vi "Receiver_Example - 2 Channel - Experiment_7.vi"() -> ()   [LabVIEW 2022 SP3]
panel:
  out "x = 0?":bool
  out "iterationsIM":dbl
  in  "State":i32
  in  "Counter":dbl
  in  "OFDM - 4QAM/16QAM":bool
  out "Iterations 2":i32
  in  "Tab Control 3":enum32{"OFDM - 4QAM", "16QAM"}(tab)
  in  "Tab Control":enum32{"USRP Parameters", "Rx Info", "BER"}(tab)
  in  "USRP ControledParameters":T1={"Active Antenna"="RX2", "Gain (dB)"=10.0, "Carrier Frequency"=2400000000.0, "IQ Rate"=2000000.0, "Active channels"="0,1"} {"IQ Rate" format="%#_6p"; "Carrier Frequency" format="%#_6p"; "Gain (dB)" format="%#_6f"}
  in  "Device selection":refnum<k15>="RIO0"
  in  "Trigger level":dbl=0.005 format="%f"
  out "CH0":T2
  out "CH1":T2
  out "SIG valid? - CH1":bool
  out "SIG valid? - CH0":bool
  out "Frequency offset - CH1":dbl
  out "Frequency offset - CH0":dbl
  out "Coerced Parameters":T3={"IQ Rate"=100000.0, "Carrier  Freq."=100000.0, "Gain"=0.0} {"Gain" format="%#_6f"; "Carrier  Freq." format="%#_6p"; "IQ Rate" format="%#_6p"}
  out "Error out":errorcluster
  in  "Expected message LP - CH0":string="Non Critical Data\nNon Critical Data\nNon Critical Data\nNon Critical Data\nNon Critical Data"
  in  "Expected message - CH1":string="Critical Dataaaaa\nCritical Dataaaaa\nCritical Dataaaaa\nCritical Dataaaaa\nCritical Dataaaaa"
  out "Expected message LP Detected CH0":string="Non Critical Data\nNon Critical Data\nNon Critical Data\nNon Critical Data\nNon Critical Data"
  out "Expected message HP Detected CH1":string="Non Critical Data\nNon Critical Data\nNon Critical Data\nNon Critical Data\nNon Critical Data"
  in  "Boolean":bool
  in  "Boolean 3":bool
  out "Expected message HP Detected CH0":string="Non Critical Data\nNon Critical Data\nNon Critical Data\nNon Critical Data\nNon Critical Data"
  in  "Expected message HP - CH0":string="Critical Dataaaaa\nCritical Dataaaaa\nCritical Dataaaaa\nCritical Dataaaaa\nCritical Dataaaaa"
  in  "Boolean 2":bool
  out "Inst. BER HP - CH0":dbl format="%#_4g"
  out "Acc. BER HP - CH0":dbl format="%#_4g"
  out "Acum. Err HP - CH0":dbl
  out "No. Bits HP - CH0":dbl
  out "Acc. BER LP - CH0":dbl format="%#_4g"
  out "Inst. BER - CH1":dbl format="%#_4g"
  out "Inst. BER LP - CH0":dbl format="%#_4g"
  out "No. Bits - CH1":dbl
  out "No. Bits LP - CH0":dbl
  out "Acum. Err - CH1":dbl
  out "Acum. Err LP - CH0":dbl
  in  "Record BER":bool
  in  "Refresh Button":bool
  out "Acc. BER - CH1":dbl format="%#_4g"
  in  "Low-Power Window Size - CH0":dbl=15.0 format="%#_6p"
  in  "High-Power Window Size":dbl=15.0 format="%#_6p"
  out "High-Power Image 2":T4(plugin-control)
  in  "Tab Control 2":enum32{"1 Channel", "2 Channel"}(tab)
  in  "Save data 1 channel":bool
  out "Constellation Map 1 Channel":cdb[](graph)
  out "Low-Power BER - 1 Channel":dbl(graph)
  out "High-Power BER - 1 Channel":dbl(graph)
  out "High-Power Decoded message - 1 Channel":string
  out "Low-Power Decoded message - 1 Channel":string
  out "Low-Power Decoded message - CH0":string
  out "Decoded message - CH1":string
  out "Constellation Map 2 Channel":cluster{"Constellation":cdb[]}[](graph)
  out "Low-Power BER - CH0":dbl(graph)
  out "High-Power BER":T5(graph)
  out "High-Power Decoded message - CH0":string
  out "CH1 2":bool
  out "CH0 2":bool
  in  "Save data 2 channels":bool
  in  "Channel":bool
  in  "Save data":bool
  out "Reconstructed Image":T4(plugin-control)
  out "Expected message  HP  Detected 2":string="Critical Dataaaaa\nCritical Dataaaaa\nCritical Dataaaaa\nCritical Dataaaaa\nCritical Dataaaaa"
  in  "Boolean 4":bool
  in  "High-Power Window Size 2":dbl=15.0 format="%#_6p"
  out "High-Power Instantaneous BER Graph 2":u8(slide) scale=0.0..100.0
  out "High-Power BER Graph 2":dbl(graph)
  out "No. Bits HP 2":dbl
  out "Acc. BER  HP 2":dbl format="%#_4g"
  out "Acum. Err HP 2":dbl
  out "Inst. BER HP 2":dbl format="%#_4g"
  in  "Expected message 2 HP 2":string="Critical Dataaaaa\nCritical Dataaaaa\nCritical Dataaaaa\nCritical Dataaaaa\nCritical Dataaaaa"
  out "High-Power Decoded Message 2":string
  in  "Record BER 2":bool
  out "Constellation Map 2":cdb[](graph)
  out "Frequency offset 2":dbl
  out "SIG valid? 2":bool
  in  "Refresh Button 2":bool
  out "Error out 2":errorcluster
  in  "error in (no error)":errorcluster
  # "OFDM Superposition Coded Receiver"
  # "1 Channel"
  # "2 Channel"
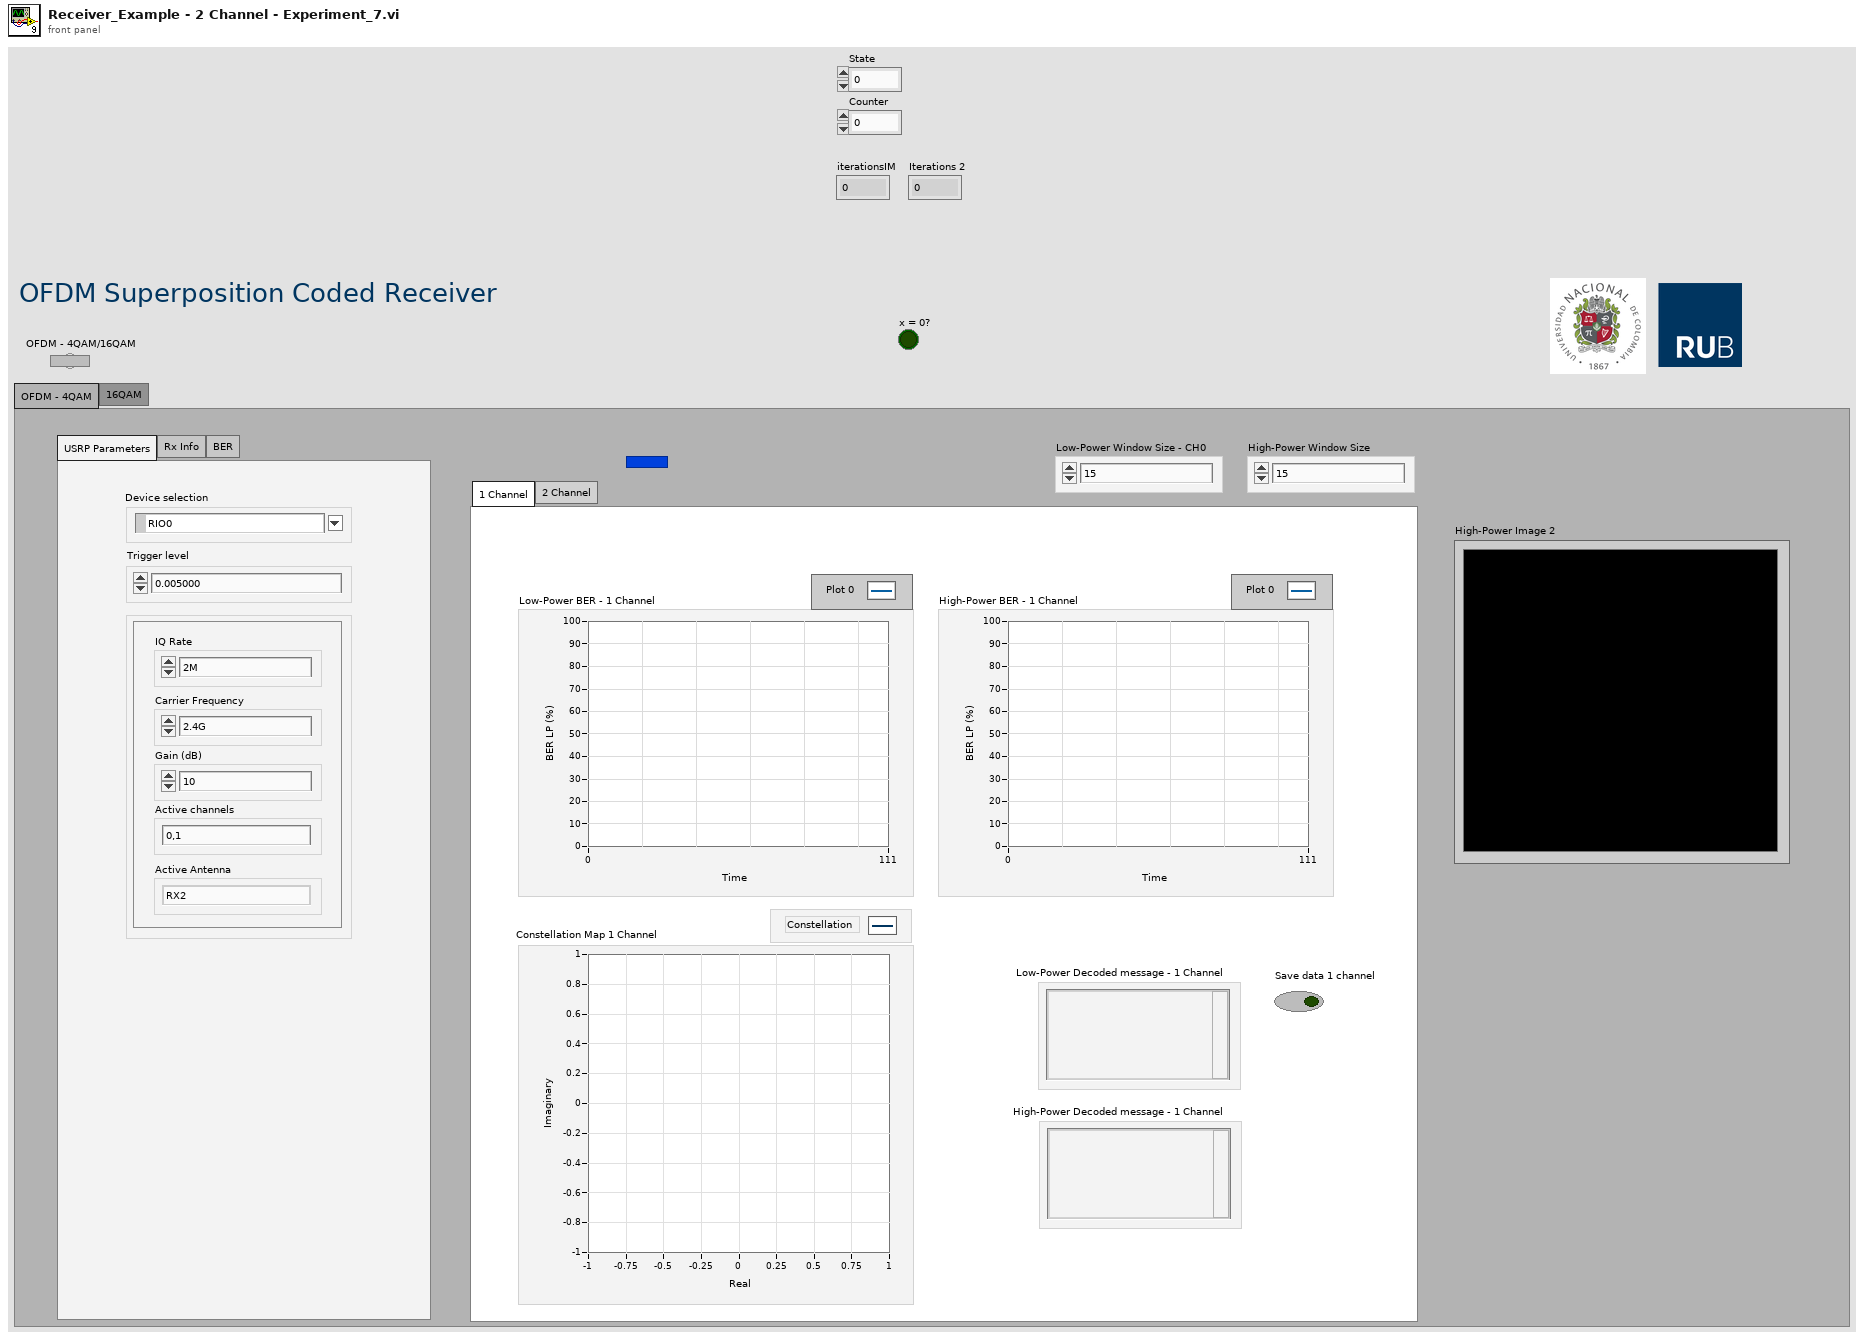
[diagram p1: front panel]
types:
  T1 = cluster{"Active Antenna":string, "Gain (dB)":dbl, "Carrier Frequency":dbl, "IQ Rate":dbl, "Active channels":string}
  T2 = cluster{"Modulation type":enum16{"QPSK(4QAM)", "64QAM", "16QAM", "BPSK"}, "BCC rate (k/n)":enum16{"1/2", "2/3", "3/4"}}
  T3 = cluster{"IQ Rate":dbl, "Carrier  Freq.":dbl, "Gain":dbl}
  T4 = typedef "IMAQ Image.ctl" = refnum<image>
  T5 = cluster{"Graph Instantaneous BER":dbl, "Graph Instantaneous BER":dbl, "Inst. BER - CH1":dbl}
  T6 = enum16{"open", "replace", "create", "open or create", "replace or create", "replace or create with confirmation"}
  T7 = cluster{"coerced IQ rate":dbl, "coerced carrier frequency":dbl, "coerced gain":dbl}
  T8 = cluster{"Graph Instantaneous BER":dbl, "Graph Instantaneous BER":dbl, "Graph Instantaneous BER":dbl}
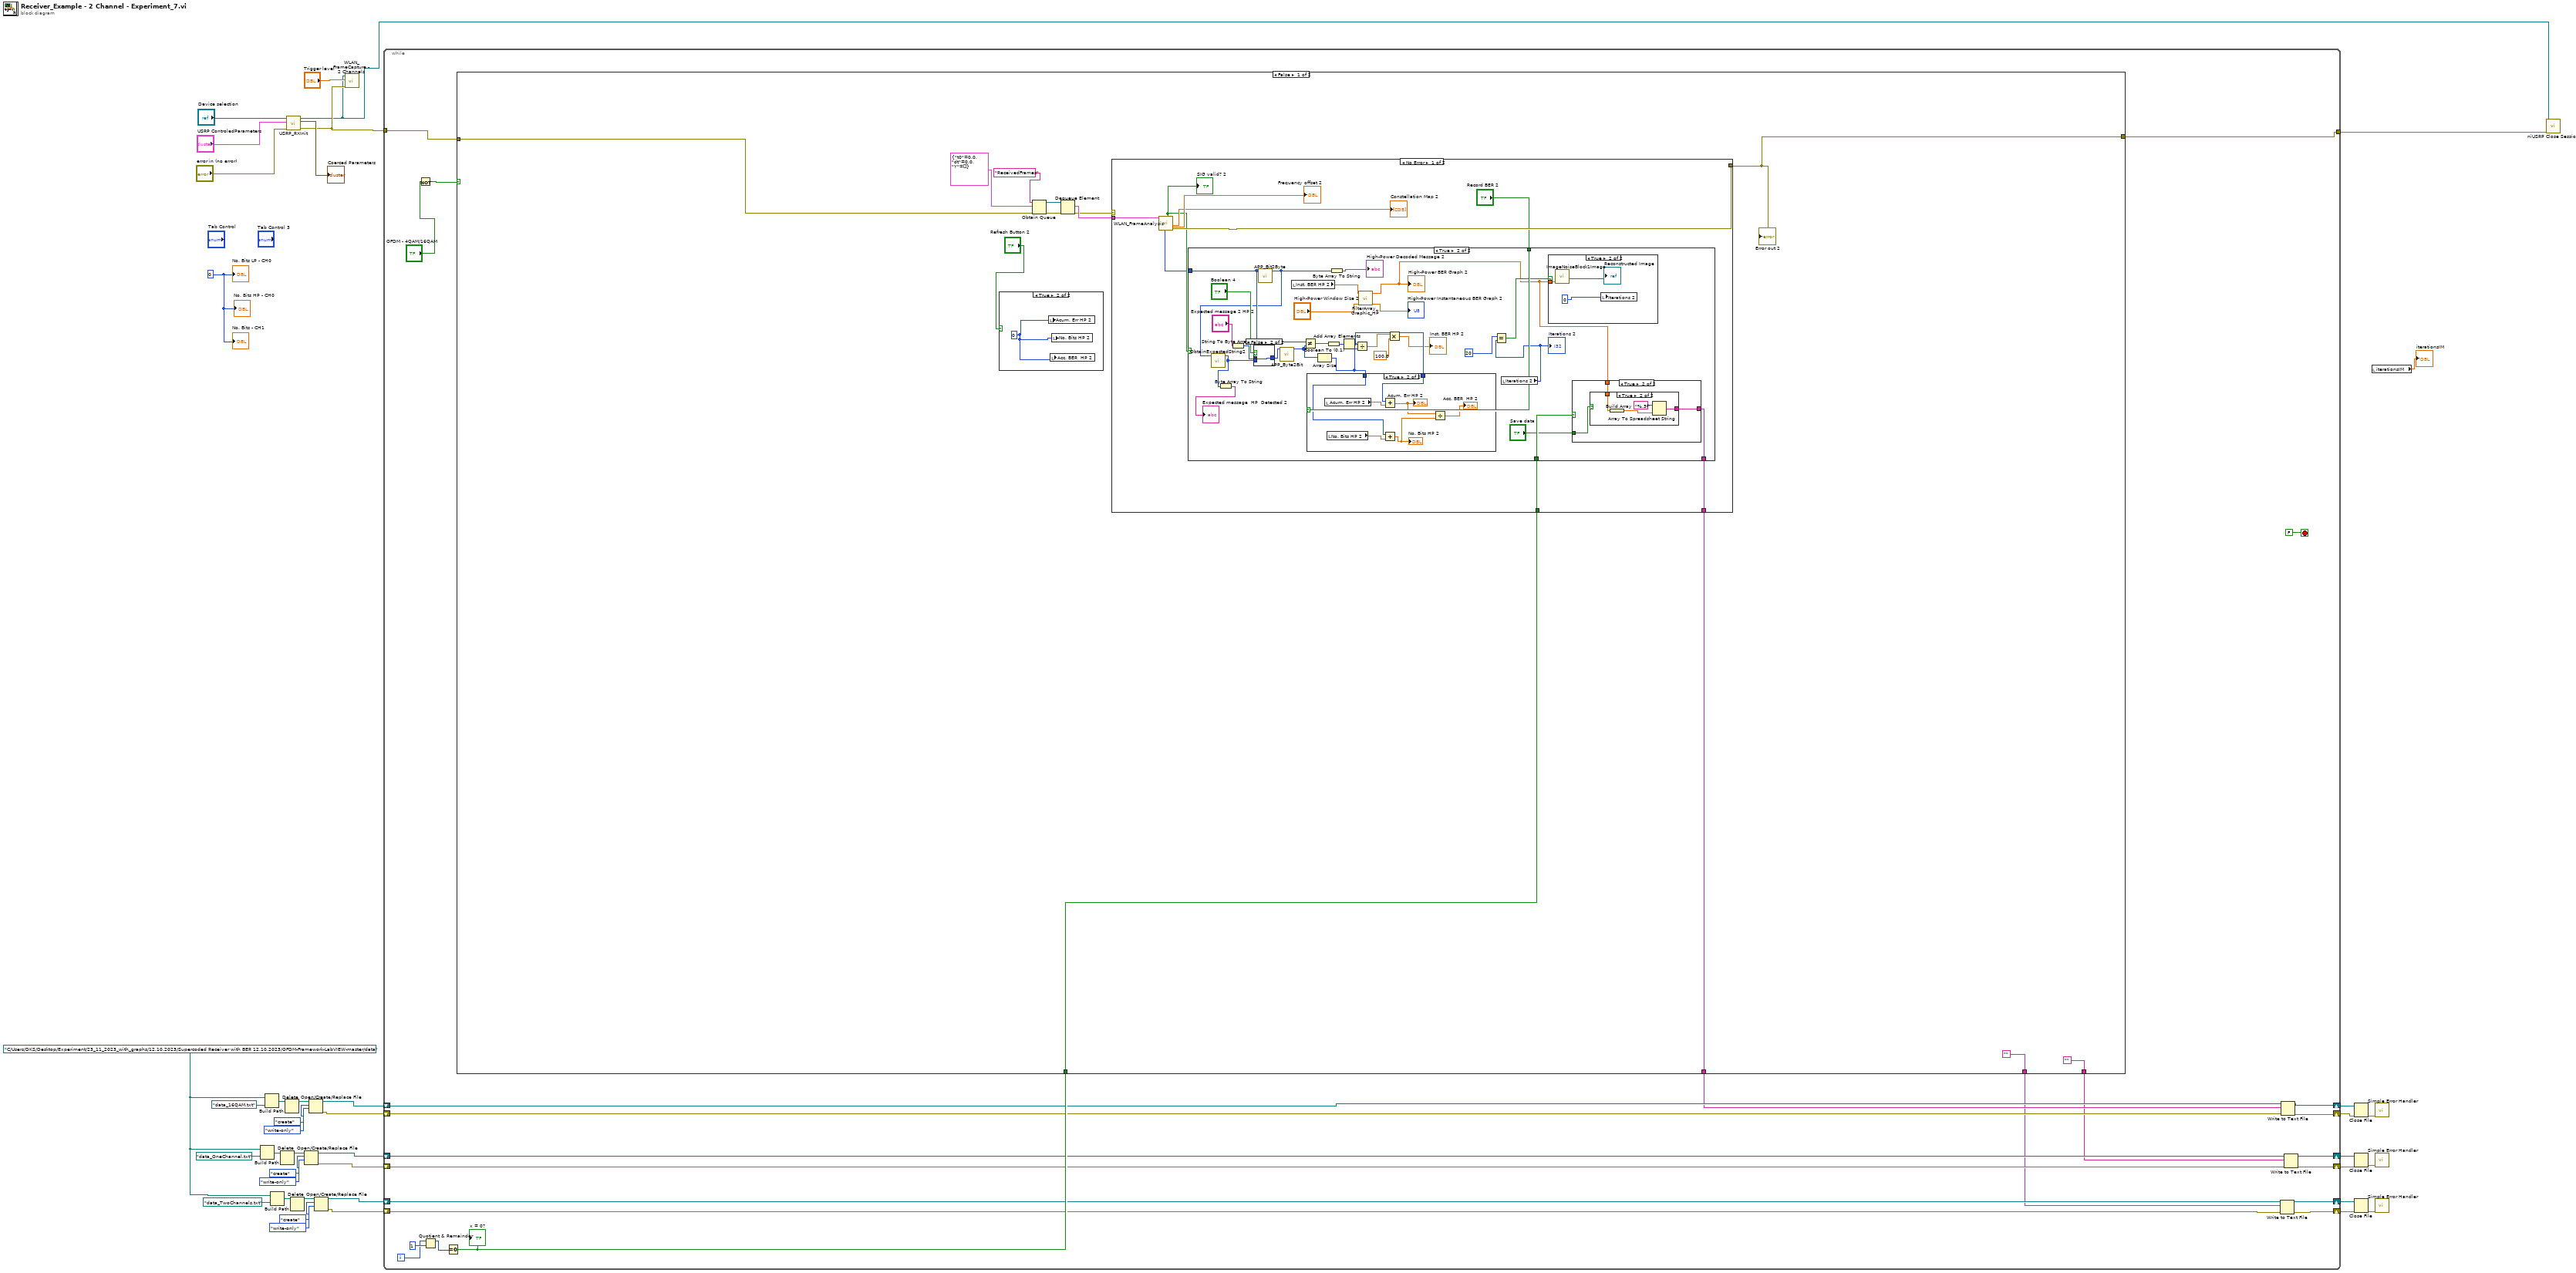
[diagram p0: block diagram]
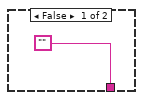
[diagram p3: hidden frame]
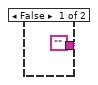
[diagram p4: hidden frame]
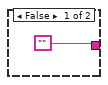
[diagram p5: hidden frame]
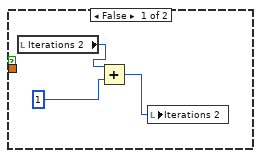
[diagram p6: hidden frame]
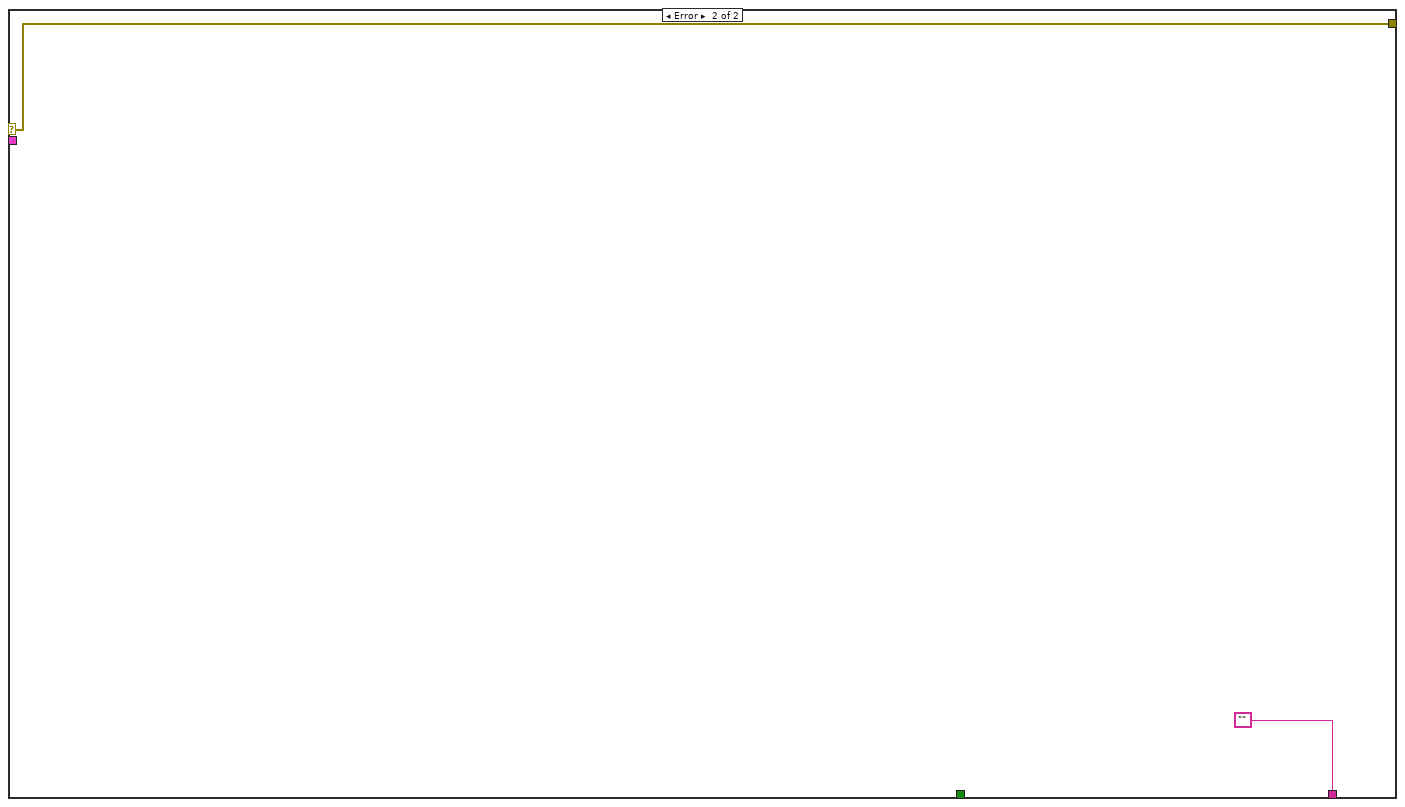
[diagram p9: hidden frame]
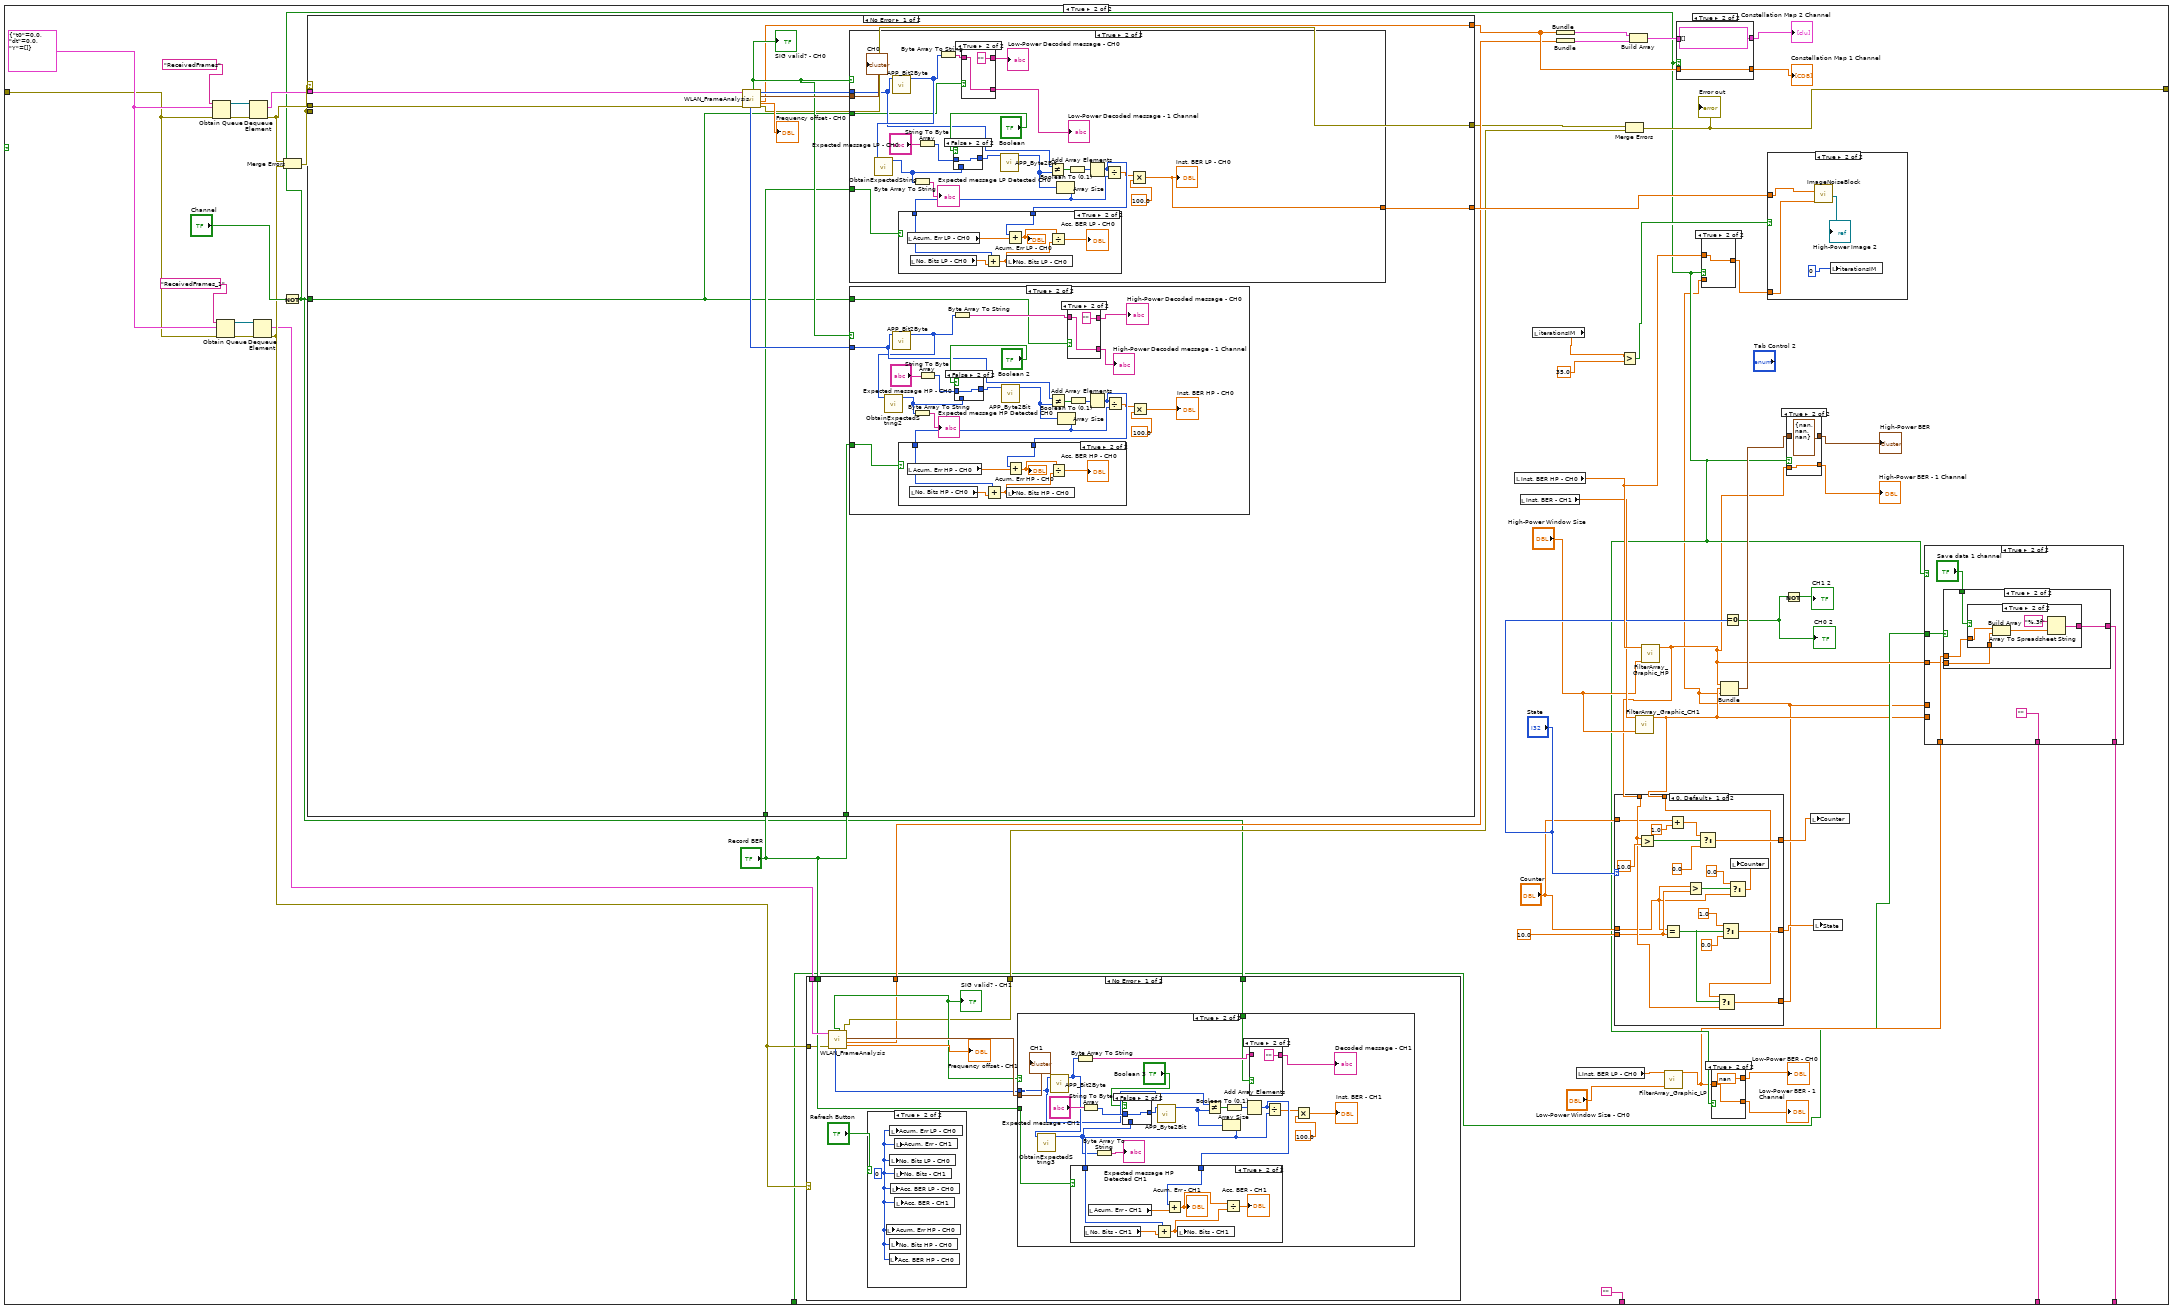
[diagram p10: hidden frame]
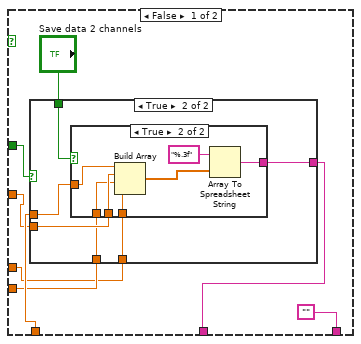
[diagram p11: hidden frame]
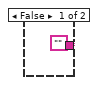
[diagram p12: hidden frame]
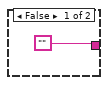
[diagram p13: hidden frame]
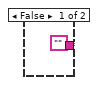
[diagram p14: hidden frame]
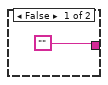
[diagram p15: hidden frame]
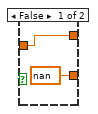
[diagram p16: hidden frame]
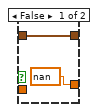
[diagram p17: hidden frame]
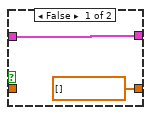
[diagram p19: hidden frame]
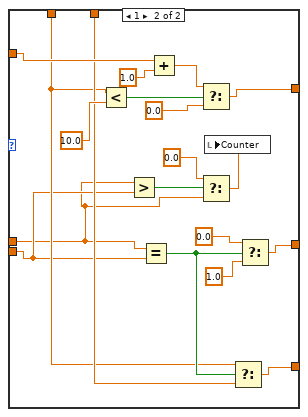
[diagram p20: hidden frame]
diagram:
  w11 = path "C:/Users/DKS/Desktop/Experiment/23_11_2023_with_graphs/12.10.2023/Supercoded Receiver with BER 12.10.2023/OFDM-Framework-LabVIEW-master/data"
  w33 = 0
  n1 = Build Path(base path=w11, name or relative path=path "data_OneChannel.txt" ("default name")) -> (appended path=w21:path)
  n2 = Build Path(base path=w11, name or relative path=path "data_16QAM.txt" ("default name")) -> (appended path=w31:path)
  n3 = Build Path(base path=w11, name or relative path=path "data_TwoChannels.txt" ("default name")) -> (appended path=w16:path)
  n4 = Delete(path (use dialog)=w21) -> (deleted path=w20:path)  [unwired: 4 in, 2 out]
  n5 = Delete(path (use dialog)=w31) -> (deleted path=w30:path)  [unwired: 4 in, 2 out]
  n6 = call "USRP_RXInit.vi"("device names"="Device selection", "USRP ControledParameters"="USRP ControledParameters", "error in (no error)"="error in (no error)") -> ("session handle out"=w36:refnum<k15>, "USRP CoercedParamters"=→"Coerced Parameters":T7, "error out"=w39:errorcluster)  [unwired: 5 in]
  n7 = Delete(path (use dialog)=w16) -> (deleted path=w15:path)  [unwired: 4 in, 2 out]
  n8 = Open/Create/Replace File(file path (use dialog)=w20, operation (0:open)=T6."create", access (0:read/write)=enum16{"read/write", "read-only", "write-only"}."write-only") -> (refnum out=w8:refnum<file>, error out=w7:errorcluster)  [unwired: 1 in, 3 out]
  n9 = Open/Create/Replace File(file path (use dialog)=w30, operation (0:open)=T6."create", access (0:read/write)=enum16{"read/write", "read-only", "write-only"}."write-only") -> (refnum out=w24:refnum<file>, error out=w25:errorcluster)  [unwired: 1 in, 3 out]
  n10 = Open/Create/Replace File(file path (use dialog)=w15, operation (0:open)=T6."create", access (0:read/write)=enum16{"read/write", "read-only", "write-only"}."write-only") -> (refnum out=w6:refnum<file>, error out=w5:errorcluster)  [unwired: 1 in, 3 out]
  n11 = call "WLAN_FrameCapture - 2 Channels.vi"("error in (no error)"=w39, "Trigger level"="Trigger level", "session handle"=w36) -> ()  [unwired: 8 in]
  n12 = while {
    tunnel: w39 -> [w65]
    tunnel: [w64] -> w37
    shift-right: [w56] -> w23
    shift-left: w25 -> [w54]
    shift-right: [w55] -> w22
    shift-left: w24 -> [w53]
    shift-right: [w50] -> w4
    shift-left: w8 -> [w51]
    shift-right: [w48] -> w3
    shift-left: w7 -> [w49]
    shift-right: [w44] -> w2
    shift-left: w6 -> [w47]
    shift-right: [w45] -> w1
    shift-left: w5 -> [w46]
    i -> [w58]
    stop <- FALSE stop-if-true
    n13 = Not(x="OFDM - 4QAM/16QAM") -> (.not. x?=w62:bool)
    n14 = Quotient & Remainder(x=w58, y=1) -> (x-y*floor(x/y)=w59:i32)  [unwired: 1 out]
    n15 = Equal To 0?(x=w59) -> (x = 0?=w57:bool)
    "x = 0?" <- w57
    n16 = case shown="False" w62 {
      tunnel: w65 -> [w71 w158]
      tunnel: [w70 w157] -> w64
      tunnel: w57 -> [w69 w148]
      tunnel: [w68 ""] -> w52
      tunnel: ["" w147] -> w43
      tunnel: ["" w144] -> w42
      frame False {
        n17 = case shown="True" "Refresh Button 2" {
          frame False {
          }
          frame True {
            w79 = 0
            n18 = local write "Acum. Err HP 2"(w79) -> ()
            n19 = local write "Acc. BER  HP 2"(w79) -> ()
            n20 = local write "No. Bits HP 2"(w79) -> ()
          }
        }
        n21 = Obtain Queue(name (unnamed)="ReceivedFrames", element data type=cluster{"t0":dbl, "dt":dbl, "Y":cdb[]} {"t0"=0.0, "dt"=0.0, "Y"=[]} ("data"), error in (no error)=w71) -> (queue out=w72:refnum<queue>, error out=w75:errorcluster)  [unwired: 2 in, 1 out]
        n22 = Dequeue Element(queue=w72, error in (no error)=w75) -> (element=w74:cluster{"t0":dbl, "dt":dbl, "Y":cdb[]}, error out=w73:errorcluster)  [unwired: 1 in, 2 out]
        n23 = case shown="No Error" w73 {
          selector: w73 -> [_ w143]
          tunnel: w74 -> [w87 _]
          tunnel: [w88 w143] -> w70
          tunnel: w69 -> [w81 _]
          tunnel: [w80 ""] -> w68
          frame No Error {
            n24 = call "WLAN_FrameAnalysis.vi"("input cluster"=w87) -> ("error out"=w88:errorcluster, "Constellation"=→"Constellation Map 2":cdb[], "Frequency offset"=→"Frequency offset 2":dbl, "SIG valid?"=w83:bool, "outputbitsHP"=w82:i8[])  [unwired: 4 in, 2 out]
            "SIG valid? 2" <- w83
            n25 = case shown="True" w83 {
              tunnel: "Record BER 2" -> [_ w111]
              tunnel: w82 -> [_ w106]
              tunnel: w81 -> [_ w92]
              tunnel: ["" w90] -> w80
              frame False {
              }
              frame True {
                n26 = String To Byte Array(string="Expected message 2 HP 2") -> (unsigned byte array=w104:u8[])
                n27 = call "APP_Bit2Byte.vi"("input bit stream"=w106) -> ("output byte stream"=w100:u8[])  [unwired: 10 in]
                n28 = call "ObtainExpectedString2.vi"("Array"=w100) -> ("detectedMessage"=w102:i8[])  [unwired: 9 in]
                n29 = Byte Array To String(unsigned byte array=w102) -> (string=→"Expected message  HP  Detected 2":string)
                n30 = case shown="False" "Boolean 4" {
                  tunnel: [w133 w134] -> w105
                  tunnel: w104 -> [_ w134]
                  tunnel: w102 -> [w133 _]
                  frame True {
                  }
                  frame False {
                  }
                }
                n31 = call "APP_Byte2Bit.vi"("input byte stream"=w105) -> ("output bit stream"=w107:i8[])  [unwired: 10 in]
                n32 = local read "Inst. BER HP 2"() -> (w110:dbl)
                n33 = Not Equal?(x=w106, y=w107) -> (x != y?=w115:bool[])
                n34 = Array Size(array=w107) -> (size(s)=w112:i32)
                n35 = Boolean To (0,1)(Boolean=w115) -> (0, 1=w114:i16[])
                n36 = Byte Array To String(unsigned byte array=w100) -> (string=→"High-Power Decoded Message 2":string)
                n37 = Add Array Elements(numeric array=w114) -> (sum=w113:i16)
                n38 = case shown="True" w111 {
                  tunnel: w113 -> [_ w140]
                  tunnel: w112 -> [_ w135]
                  frame False {
                  }
                  frame True {
                    n39 = local read "Acum. Err HP 2"() -> (w141:dbl)
                    n40 = local read "No. Bits HP 2"() -> (w137:dbl)
                    n41 = Add(x=w140, y=w141) -> (x+y=w139:dbl)
                    "Acum. Err HP 2" <- w139
                    n42 = Add(x=w135, y=w137) -> (x+y=w136:dbl)
                    "No. Bits HP 2" <- w136
                    n43 = Divide(x=w139, y=w136) -> (x/y=→"Acc. BER  HP 2":dbl)
                  }
                }
                n44 = Divide(x=w113, y=w112) -> (x/y=w99:dbl)
                n45 = call "FilterArray_Graphic_HP.vi"("Window Size"="High-Power Window Size 2", "Instantaneous BER"=w110) -> ("Slide Bar"=→"High-Power Instantaneous BER Graph 2":dbl, "Graph Instantaneous BER"=w93:dbl)  [unwired: 4 in]
                "High-Power BER Graph 2" <- w93
                n46 = Multiply(x=w99, y=100.0) -> (x*y=→"Inst. BER HP 2":dbl)
                n47 = local read "Iterations 2"() -> (w95:i32)
                "Iterations 2" <- w95
                n48 = Equal?(x=20, y=w95) -> (x = y?=w94:bool)
                n49 = case shown="True" w94 {
                  tunnel: w93 -> [_ w132]
                  frame False {
                    n50 = local read "Iterations 2"() -> (w129:i32)
                    n51 = Add(x=w129, y=1) -> (x+y=w127:i32)
                    n52 = local write "Iterations 2"(w127) -> ()
                  }
                  frame True {
                    n53 = call "ImageNoiseBlock1Image.vi"("BERHP"=w132) -> ("High-Power Image"=→"Reconstructed Image":T4)  [unwired: 9 in]
                    n54 = local write "Iterations 2"(0) -> ()
                  }
                }
                n55 = case shown="True" w92 {
                  tunnel: ["" w121] -> w90
                  tunnel: w93 -> [_ w120]
                  tunnel: "Save data" -> [_ w119]
                  frame False {
                  }
                  frame True {
                    n56 = case shown="True" w119 {
                      tunnel: ["" w124] -> w121
                      tunnel: w120 -> [_ w123]
                      frame False {
                      }
                      frame True {
                        n57 = Build Array(w123) -> (w126:dbl[])
                        n58 = Array To Spreadsheet String(array=w126, 3:"%.3f") -> (spreadsheet string=w124:string)  [unwired: 1 out]
                      }
                    }
                  }
                }
              }
            }
          }
          frame Error {
          }
        }
        "Error out 2" <- w70
      }
      frame True {
        w199 = cluster{"t0":dbl, "dt":dbl, "Y":cdb[]} {"t0"=0.0, "dt"=0.0, "Y"=[]} ("data")
        n59 = Obtain Queue(name (unnamed)="ReceivedFrames", element data type=w199, error in (no error)=w158) -> (queue out=w159:refnum<queue>, error out=w161:errorcluster)  [unwired: 2 in, 1 out]
        n60 = Obtain Queue(name (unnamed)="ReceivedFrames_1", element data type=w199, error in (no error)=w158) -> (queue out=w163:refnum<queue>, error out=w164:errorcluster)  [unwired: 2 in, 1 out]
        n61 = Dequeue Element(queue=w159, error in (no error)=w161) -> (element=w160:cluster{"t0":dbl, "dt":dbl, "Y":cdb[]}, error out=w167:errorcluster)  [unwired: 1 in, 2 out]
        n62 = Dequeue Element(queue=w163, error in (no error)=w164) -> (element=w172:cluster{"t0":dbl, "dt":dbl, "Y":cdb[]}, error out=w176:errorcluster)  [unwired: 1 in, 2 out]
        n63 = Not(x="Channel") -> (.not. x?=w151:bool)
        n64 = Merge Errors(w167, w176) -> (w166:errorcluster)
        n65 = case shown="No Error" w166 {
          tunnel: w160 -> [w354 _]
          tunnel: w166 -> [_ w429]
          tunnel: w167 -> [w351 _]
          tunnel: [w350 100] -> w178
          tunnel: [w349 dbl[] []] -> w189
          tunnel: [w348 w429] -> w173
          tunnel: "Record BER" -> [w347 _]
          tunnel: "Record BER" -> [w346 _]
          tunnel: w151 -> [w345 _]
          frame No Error {
            n66 = call "WLAN_FrameAnalysis.vi"("error in (no error)"=w351, "input cluster"=w354) -> ("error out"=w348:errorcluster, "Constellation"=w349:cdb[], "Modulation parameter"=w355:T2, "output bits"=w356:i8[], "Frequency offset"=→"Frequency offset - CH0":dbl, "SIG valid?"=w352:bool, "outputbitsHP"=w353:i8[])  [unwired: 3 in]
            "SIG valid? - CH0" <- w352
            n67 = case shown="True" w352 {
              tunnel: w356 -> [_ w398]
              tunnel: w355 -> [_ w414]
              tunnel: w346 -> [_ w410]
              tunnel: [100.0 w397] -> w350
              tunnel: w345 -> [_ w393]
              frame False {
              }
              frame True {
                n68 = call "APP_Bit2Byte.vi"("input bit stream"=w398) -> ("output byte stream"=w402:u8[])  [unwired: 10 in]
                n69 = call "ObtainExpectedString.vi"("Array"=w402) -> ("detectedMessage"=w399:i8[])  [unwired: 9 in]
                n70 = Byte Array To String(unsigned byte array=w399) -> (string=→"Expected message LP Detected CH0":string)
                n71 = String To Byte Array(string="Expected message LP - CH0") -> (unsigned byte array=w403:u8[])
                n72 = Byte Array To String(unsigned byte array=w402) -> (string=w396:string)
                n73 = case shown="False" "Boolean" {
                  tunnel: [w419 w420] -> w405
                  tunnel: w403 -> [_ w420]
                  tunnel: w399 -> [w419 _]
                  frame True {
                  }
                  frame False {
                  }
                }
                n74 = case shown="True" w393 {
                  tunnel: w396 -> [w416 w418]
                  tunnel: ["" ("string") w418] -> w395
                  tunnel: [w416 "" ("string")] -> w394
                  frame False {
                  }
                  frame True {
                  }
                }
                "Low-Power Decoded message - CH0" <- w394
                "Low-Power Decoded message - 1 Channel" <- w395
                n75 = call "APP_Byte2Bit.vi"("input byte stream"=w405) -> ("output bit stream"=w404:i8[])  [unwired: 10 in]
                n76 = Not Equal?(x=w398, y=w404) -> (x != y?=w412:bool[])
                n77 = Array Size(array=w404) -> (size(s)=w409:i32)
                n78 = Boolean To (0,1)(Boolean=w412) -> (0, 1=w413:i16[])
                n79 = Add Array Elements(numeric array=w413) -> (sum=w408:i16)
                n80 = case shown="True" w410 {
                  tunnel: w409 -> [_ w426]
                  tunnel: w408 -> [_ w424]
                  frame False {
                  }
                  frame True {
                    n81 = local read "Acum. Err LP - CH0"() -> (w425:dbl)
                    n82 = local read "No. Bits LP - CH0"() -> (w427:dbl)
                    n83 = Add(x=w426, y=w427) -> (x+y=w423:dbl)
                    n84 = Add(x=w424, y=w425) -> (x+y=w422:dbl)
                    "Acum. Err LP - CH0" <- w422
                    n85 = local write "No. Bits LP - CH0"(w423) -> ()
                    n86 = Divide(x=w422, y=w423) -> (x/y=→"Acc. BER LP - CH0":dbl)
                  }
                }
                n87 = Divide(x=w408, y=w409) -> (x/y=w407:dbl)
                n88 = Multiply(x=w407, y=100.0) -> (x*y=w397:dbl)
                "Inst. BER LP - CH0" <- w397
                "CH0" <- w414
              }
            }
            n89 = case shown="True" w352 {
              tunnel: w353 -> [_ w365]
              tunnel: w347 -> [_ w375]
              tunnel: w345 -> [_ w358]
              frame False {
              }
              frame True {
                n90 = call "APP_Bit2Byte.vi"("input bit stream"=w365) -> ("output byte stream"=w364:u8[])  [unwired: 10 in]
                n91 = call "ObtainExpectedString2.vi"("Array"=w364) -> ("detectedMessage"=w363:i8[])  [unwired: 9 in]
                n92 = Byte Array To String(unsigned byte array=w363) -> (string=→"Expected message HP Detected CH0":string)
                n93 = String To Byte Array(string="Expected message HP - CH0") -> (unsigned byte array=w368:u8[])
                n94 = Byte Array To String(unsigned byte array=w364) -> (string=w359:string)
                n95 = case shown="False" "Boolean 2" {
                  tunnel: [w383 w384] -> w370
                  tunnel: w368 -> [_ w384]
                  tunnel: w363 -> [w383 _]
                  frame True {
                  }
                  frame False {
                  }
                }
                n96 = call "APP_Byte2Bit.vi"("input byte stream"=w370) -> ("output bit stream"=w369:i8[])  [unwired: 10 in]
                n97 = Not Equal?(x=w365, y=w369) -> (x != y?=w377:bool[])
                n98 = Array Size(array=w369) -> (size(s)=w374:i32)
                n99 = case shown="True" w358 {
                  tunnel: w359 -> [w380 w382]
                  tunnel: ["" ("string") w382] -> w360
                  tunnel: [w380 "" ("string")] -> w361
                  frame False {
                  }
                  frame True {
                  }
                }
                "High-Power Decoded message - CH0" <- w361
                "High-Power Decoded message - 1 Channel" <- w360
                n100 = Boolean To (0,1)(Boolean=w377) -> (0, 1=w378:i16[])
                n101 = Add Array Elements(numeric array=w378) -> (sum=w373:i16)
                n102 = case shown="True" w375 {
                  tunnel: w374 -> [_ w390]
                  tunnel: w373 -> [_ w388]
                  frame False {
                  }
                  frame True {
                    n103 = local read "Acum. Err HP - CH0"() -> (w389:dbl)
                    n104 = local read "No. Bits HP - CH0"() -> (w391:dbl)
                    n105 = Add(x=w390, y=w391) -> (x+y=w387:dbl)
                    n106 = local write "No. Bits HP - CH0"(w387) -> ()
                    n107 = Add(x=w388, y=w389) -> (x+y=w386:dbl)
                    "Acum. Err HP - CH0" <- w386
                    n108 = Divide(x=w386, y=w387) -> (x/y=→"Acc. BER HP - CH0":dbl)
                  }
                }
                n109 = Divide(x=w373, y=w374) -> (x/y=w372:dbl)
                n110 = Multiply(x=w372, y=100.0) -> (x*y=→"Inst. BER HP - CH0":dbl)
              }
            }
          }
          frame Error {
            (unwired) 100
          }
        }
        n111 = case shown="No Error" w176 {
          tunnel: w172 -> [w298 _]
          tunnel: "Record BER" -> [w296 _]
          tunnel: [w295 w337] -> w174
          tunnel: [w294 dbl[] []] -> w175
          tunnel: w176 -> [w293 w337]
          tunnel: w151 -> [w292 _]
          frame No Error {
            n112 = call "WLAN_FrameAnalysis.vi"("error in (no error)"=w293, "input cluster"=w298) -> ("error out"=w295:errorcluster, "Constellation"=w294:cdb[], "Modulation parameter"=w301:T2, "Frequency offset"=→"Frequency offset - CH1":dbl, "SIG valid?"=w297:bool, "outputbitsHP"=w299:i8[])  [unwired: 3 in, 1 out]
            "SIG valid? - CH1" <- w297
            n113 = case shown="True" "Refresh Button" {
              frame False {
              }
              frame True {
                w303 = 0
                n114 = local write "Acum. Err HP - CH0"(w303) -> ()
                n115 = local write "Acc. BER HP - CH0"(w303) -> ()
                n116 = local write "Acum. Err LP - CH0"(w303) -> ()
                n117 = local write "No. Bits LP - CH0"(w303) -> ()
                n118 = local write "No. Bits HP - CH0"(w303) -> ()
                n119 = local write "Acc. BER LP - CH0"(w303) -> ()
                n120 = local write "Acum. Err - CH1"(w303) -> ()
                n121 = local write "No. Bits - CH1"(w303) -> ()
                n122 = local write "Acc. BER - CH1"(w303) -> ()
              }
            }
            n123 = case shown="True" w297 {
              tunnel: w299 -> [_ w310]
              tunnel: w301 -> [_ w324]
              tunnel: w296 -> [_ w307]
              tunnel: w292 -> [_ w304]
              frame False {
              }
              frame True {
                n124 = call "APP_Bit2Byte.vi"("input bit stream"=w310) -> ("output byte stream"=w313:u8[])  [unwired: 10 in]
                n125 = call "ObtainExpectedString3.vi"("Array"=w313) -> ("detectedMessage"=w312:i8[])  [unwired: 9 in]
                n126 = Byte Array To String(unsigned byte array=w313) -> (string=w305:string)
                n127 = String To Byte Array(string="Expected message - CH1") -> (unsigned byte array=w314:u8[])
                n128 = Byte Array To String(unsigned byte array=w312) -> (string=→"Expected message HP Detected CH1":string)
                n129 = case shown="False" "Boolean 3" {
                  tunnel: [w327 w328] -> w316
                  tunnel: w314 -> [_ w328]
                  tunnel: w312 -> [w327 _]
                  frame True {
                  }
                  frame False {
                  }
                }
                n130 = call "APP_Byte2Bit.vi"("input byte stream"=w316) -> ("output bit stream"=w315:i8[])  [unwired: 10 in]
                n131 = Not Equal?(x=w310, y=w315) -> (x != y?=w322:bool[])
                n132 = Array Size(array=w315) -> (size(s)=w320:i32)
                n133 = Boolean To (0,1)(Boolean=w322) -> (0, 1=w323:i16[])
                n134 = Add Array Elements(numeric array=w323) -> (sum=w319:i16)
                n135 = case shown="True" w307 {
                  tunnel: w320 -> [_ w334]
                  tunnel: w319 -> [_ w332]
                  frame False {
                  }
                  frame True {
                    n136 = local read "No. Bits - CH1"() -> (w335:dbl)
                    n137 = local read "Acum. Err - CH1"() -> (w333:dbl)
                    n138 = Add(x=w334, y=w335) -> (x+y=w331:dbl)
                    n139 = Add(x=w332, y=w333) -> (x+y=w330:dbl)
                    "Acum. Err - CH1" <- w330
                    n140 = local write "No. Bits - CH1"(w331) -> ()
                    n141 = Divide(x=w330, y=w331) -> (x/y=→"Acc. BER - CH1":dbl)
                  }
                }
                n142 = case shown="True" w304 {
                  tunnel: w305 -> [w325 _]
                  tunnel: [w325 "" ("string")] -> w306
                  frame False {
                  }
                  frame True {
                  }
                }
                "Decoded message - CH1" <- w306
                n143 = Divide(x=w319, y=w320) -> (x/y=w317:dbl)
                n144 = Multiply(x=w317, y=100.0) -> (x*y=→"Inst. BER - CH1":dbl)
                "CH1" <- w324
              }
            }
          }
          frame Error {
          }
        }
        n145 = local read "Inst. BER HP - CH0"() -> (w194:dbl)
        n146 = local read "Inst. BER - CH1"() -> (w184:dbl)
        n147 = local read "iterationsIM"() -> (w168:dbl)
        n148 = Bundle("Constellation"=w189) -> (w188:cluster{"Constellation":cdb[]})  [unwired: 1 in]
        n149 = Bundle("Constellation"=w175) -> (w171:cluster{"Constellation":cdb[]})  [unwired: 1 in]
        n150 = local read "Inst. BER LP - CH0"() -> (w153:dbl)
        n151 = Greater?(x=w168, y=35.0) -> (0:w169:bool)
        n152 = Merge Errors(w173, w174) -> (w157:errorcluster)
        "Error out" <- w157
        n153 = Build Array(w188, w171) -> (w191:cluster{"Constellation":cdb[]}[])
        n154 = call "FilterArray_Graphic_CH1.vi"("Window Size"="High-Power Window Size", "Instantaneous BER"=w184) -> ("Graph Instantaneous BER"=w146:dbl)  [unwired: 4 in, 1 out]
        n155 = call "FilterArray_Graphic_HP.vi"("Window Size"="High-Power Window Size", "Instantaneous BER"=w194) -> ("Graph Instantaneous BER"=w149:dbl)  [unwired: 4 in, 1 out]
        n156 = case shown="0, Default" "State" {
          tunnel: "Counter" -> [w260 w280]
          tunnel: [w267 w283] -> w180
          tunnel: "Counter" -> [w255 w273]
          tunnel: [w264 w282] -> w181
          tunnel: [w262 w281] -> w145
          tunnel: w149 -> [w261 w278]
          tunnel: w146 -> [w259 w279]
          tunnel: 10.0 ("y") -> [w258 w274]
          frame 0, Default {
            n157 = Greater?(x=w261, y=10.0) -> (0:w268:bool)
            n158 = Equal?(x=w255, y=w258) -> (x = y?=w263:bool)
            n159 = Add(x=w260, y=1.0) -> (x+y=w270:dbl)
            n160 = Greater?(x=w255, y=w258) -> (0:w257:bool)
            n161 = Select(t=w270, s=w268, f=0.0) -> (s? t:f=w267:dbl)
            n162 = Select(t=w259, s=w263, f=w261) -> (s? t:f=w262:dbl)
            n163 = Select(t=1.0, s=w263, f=0.0) -> (s? t:f=w264:dbl)
            n164 = Select(t=0.0, s=w257, f=w255) -> (s? t:f=w254:dbl)
            n165 = local write "Counter"(w254) -> ()
          }
          frame 1 {
            n166 = Less?(x=w278, y=10.0) -> (x < y?=w284:bool)
            n167 = Greater?(x=w273, y=w274) -> (0:w276:bool)
            n168 = Equal?(x=w273, y=w274) -> (x = y?=w286:bool)
            n169 = Add(x=w280, y=1.0) -> (x+y=w290:dbl)
            n170 = Select(t=w290, s=w284, f=0.0) -> (s? t:f=w283:dbl)
            n171 = Select(t=0.0, s=w276, f=w273) -> (s? t:f=w277:dbl)
            n172 = local write "Counter"(w277) -> ()
            n173 = Select(t=w278, s=w286, f=w279) -> (s? t:f=w281:dbl)
            n174 = Select(t=0.0, s=w286, f=1.0) -> (s? t:f=w282:dbl)
          }
        }
        n175 = call "FilterArray_Graphic_LP.vi"("Window Size"="Low-Power Window Size - CH0", "Instantaneous BER"=w153) -> ("Graph Instantaneous BER"=w150:dbl)  [unwired: 4 in, 1 out]
        n176 = case shown="True" w151 {
          tunnel: [cdb[] [] ("Constellation") w253] -> w190
          tunnel: w189 -> [_ w253]
          tunnel: w191 -> [w251 _]
          tunnel: [w251 cluster{"Constellation":cdb[]}[] []] -> w192
          frame False {
          }
          frame True {
          }
        }
        "Constellation Map 2 Channel" <- w192
        "Constellation Map 1 Channel" <- w190
        n177 = case shown="True" w151 {
          tunnel: w194 -> [_ w249]
          tunnel: [w248 w249] -> w195
          tunnel: w145 -> [w248 _]
          frame False {
          }
          frame True {
          }
        }
        n178 = case shown="True" w151 {
          tunnel: w150 -> [w241 w243]
          tunnel: [nan ("Graph Instantaneous BER") w243] -> w154
          tunnel: [w241 nan ("Graph Instantaneous BER")] -> w155
          frame False {
          }
          frame True {
          }
        }
        "Low-Power BER - CH0" <- w155
        "Low-Power BER - 1 Channel" <- w154
        n179 = Bundle("Graph Instantaneous BER"=w149, "Graph Instantaneous BER"=w146, "Graph Instantaneous BER"=w145) -> (w197:T8)  [unwired: 1 in]
        n180 = Equal To 0?(x="State") -> (x = 0?=w187:bool)
        "CH0 2" <- w187
        n181 = case shown="True" w169 {
          tunnel: w195 -> [_ w344]
          tunnel: w178 -> [_ w341]
          frame False {
            n182 = local read "iterationsIM"() -> (w340:dbl)
            n183 = Add(x=1, y=w340) -> (x+y=w339:dbl)
            n184 = local write "iterationsIM"(w339) -> ()
          }
          frame True {
            n185 = call "ImageNoiseBlock.vi"("BERLP"=w341, "BERHP"=w344) -> ("High-Power Image"=→"High-Power Image 2":T4)  [unwired: 8 in]
            n186 = local write "iterationsIM"(0) -> ()
          }
        }
        n187 = Not(x=w187) -> (.not. x?=→"CH1 2":bool)
        n188 = case shown="True" w151 {
          tunnel: w149 -> [_ w247]
          tunnel: [nan w247] -> w196
          tunnel: w197 -> [w245 _]
          tunnel: [w245 T8 {"Graph Instantaneous BER"=nan, "Graph Instantaneous BER"=nan, "Graph Instantaneous BER"=nan}] -> w198
          frame False {
          }
          frame True {
          }
        }
        "High-Power BER" <- w198
        "High-Power BER - 1 Channel" <- w196
        n189 = local write "Counter"(w180) -> ()
        n190 = local write "State"(w181) -> ()
        n191 = case shown="True" w151 {
          tunnel: w150 -> [w204 w228]
          tunnel: w149 -> [w203 w227]
          tunnel: w148 -> [w206 w226]
          tunnel: ["" w224] -> w147
          tunnel: w146 -> [w202 _]
          tunnel: w145 -> [w201 _]
          tunnel: [w200 ""] -> w144
          frame False {
            n192 = case shown="True" w206 {
              tunnel: ["" w214] -> w200
              tunnel: w204 -> [_ w212]
              tunnel: w203 -> [_ w213]
              tunnel: "Save data 2 channels" -> [_ w211]
              tunnel: w202 -> [_ w210]
              tunnel: w201 -> [_ w209]
              frame False {
              }
              frame True {
                n193 = case shown="True" w211 {
                  tunnel: ["" w220] -> w214
                  tunnel: w212 -> [_ w219]
                  tunnel: w213 -> [_ w218]
                  tunnel: w210 -> [_ w217]
                  tunnel: w209 -> [_ w216]
                  frame False {
                  }
                  frame True {
                    n194 = Build Array(w219, w218, w217, w216) -> (w222:dbl[])
                    n195 = Array To Spreadsheet String(array=w222, 3:"%.3f") -> (spreadsheet string=w220:string)  [unwired: 1 out]
                  }
                }
              }
            }
          }
          frame True {
            n196 = case shown="True" w226 {
              tunnel: ["" w233] -> w224
              tunnel: w228 -> [_ w231]
              tunnel: w227 -> [_ w232]
              tunnel: "Save data 1 channel" -> [_ w230]
              frame False {
              }
              frame True {
                n197 = case shown="True" w230 {
                  tunnel: ["" w237] -> w233
                  tunnel: w231 -> [_ w236]
                  tunnel: w232 -> [_ w235]
                  frame False {
                  }
                  frame True {
                    n198 = Build Array(w236, w235) -> (w239:dbl[])
                    n199 = Array To Spreadsheet String(array=w239, 3:"%.3f") -> (spreadsheet string=w237:string)  [unwired: 1 out]
                  }
                }
              }
            }
          }
        }
      }
    }
    n200 = Write to Text File(file (use dialog)=w47, text=w42, error in=w46) -> (refnum out=w44:refnum<file>, error out=w45:errorcluster)  [unwired: 1 in, 1 out]
    n201 = Write to Text File(file (use dialog)=w53, text=w52, error in=w54) -> (refnum out=w55:refnum<file>, error out=w56:errorcluster)  [unwired: 1 in, 1 out]
    n202 = Write to Text File(file (use dialog)=w51, text=w43, error in=w49) -> (refnum out=w50:refnum<file>, error out=w48:errorcluster)  [unwired: 1 in, 1 out]
  }
  n203 = Close File(refnum=w22, error in=w23) -> (error out=w26:errorcluster)  [unwired: 1 out]
  n204 = Close File(refnum=w4, error in=w3) -> (error out=w10:errorcluster)  [unwired: 1 out]
  n205 = Close File(refnum=w2, error in=w1) -> (error out=w9:errorcluster)  [unwired: 1 out]
  n206 = local read "iterationsIM"() -> (→"iterationsIM":dbl)
  n207 = call <vilib>:"Simple Error Handler.vi"("error in (no error)"=w26) -> ()  [unwired: 1 in, 8 out]
  n208 = call <vilib>:"Simple Error Handler.vi"("error in (no error)"=w10) -> ()  [unwired: 1 in, 8 out]
  n209 = call <vilib>:"Simple Error Handler.vi"("error in (no error)"=w9) -> ()  [unwired: 1 in, 8 out]
  n210 = call <instrlib>:"niUSRP Close Session.vi"("session handle"=w36, "error in (no error)"=w37) -> ()  [unwired: 13 in, 1 out]
  "No. Bits LP - CH0" <- w33
  "No. Bits - CH1" <- w33
  "No. Bits HP - CH0" <- w33
